vi "Extract Depth Param.vi"(1 "Eye Model Cluster":T2={"X Grid"=[], "Y Grid"=[], "Za_true Surf"=[], "Iris Center"=[0.0, 5.0, 0.0], "Zp_true Surf"=[], "Pinv"=[[1.0, 0.0], [0.0, 1.0]], "za_true"=2.0, "za_work"=1.0, "zp_work"=-1.0, "zp_true"=-2.0}) -> (0 "Nominal Model param":T3={"za_true_0"=2.0, "za_work_0"=1.0, "zp_work_0"=-1.0, "zp_true_0"=-2.0, "IrisCenter_0"=[0.0, 5.0, 0.0]})   [LabVIEW 2016]
uses:
  <vilib>/Analysis/Matrix/Datatypes/RealMatrix.ctl
  <vilib>/Analysis/Matrix/NI_Matrix.lvlib
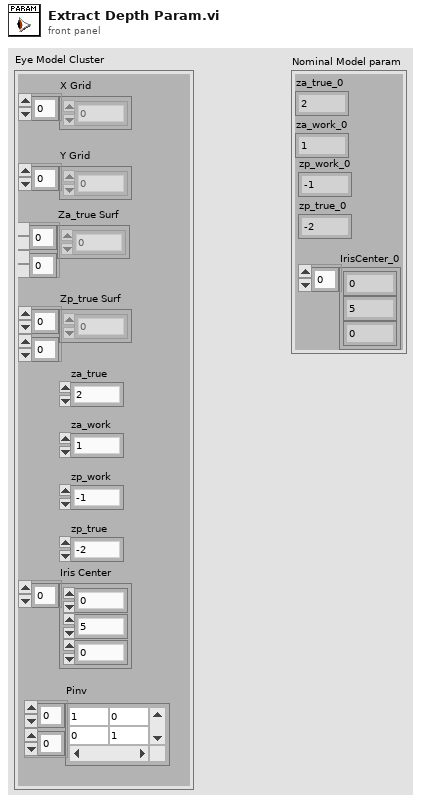
[diagram p1: front panel]
types:
  T1 = typedef "NI_Matrix.lvlib/RealMatrix.ctl" = dbl[][]
  T2 = cluster{"X Grid":dbl[], "Y Grid":dbl[], "Za_true Surf":dbl[][], "Iris Center":dbl[], "Zp_true Surf":dbl[][], "Pinv":T1, "za_true":dbl, "za_work":dbl, "zp_work":dbl, "zp_true":dbl}
  T3 = cluster{"za_true_0":dbl, "za_work_0":dbl, "zp_work_0":dbl, "zp_true_0":dbl, "IrisCenter_0":dbl[]}
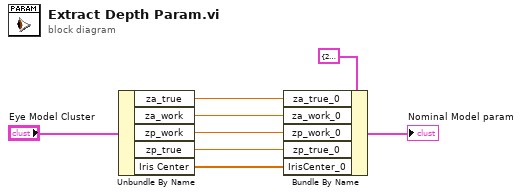
[diagram p0: block diagram]
diagram:
  n1 = Unbundle By Name("Eye Model Cluster") -> ("za_true"=w5:dbl, "za_work"=w4:dbl, "zp_work"=w3:dbl, "zp_true"=w2:dbl, "Iris Center"=w1:dbl[])
  n2 = Bundle By Name(cluster=T3 {"za_true_0"=2.0, "za_work_0"=1.0, "zp_work_0"=-1.0, "zp_true_0"=-2.0, "IrisCenter_0"=[0.0, 5.0, 0.0]} ("Nominal Model param"), "za_true_0"=w5, "za_work_0"=w4, "zp_work_0"=w3, "zp_true_0"=w2, "IrisCenter_0"=w1) -> (→"Nominal Model param":T3)
